vi "Process.vi"(8 "error in":errorcluster, 11 "SignalReceiver":refnum<class "SignalReceiver.lvclass">) -> (0 "error out":errorcluster, 3 "SignalReceiver out":refnum<class "SignalReceiver.lvclass">)   [LabVIEW 2020, in "ECU_Diagnose.lvlib" / "SignalReceiver.lvclass"]
doc: "---------------------------------------------------------------\nJKI State Machine Objects™\nhttp://jki.net/state-machine-objects/\nCopyright (C) 2005-2015, JKI <info@jki.net>\nALL RIGHTS RESERVEDJKI State Machine Objects (SMO) 1.0.0.5\nJKI - JKI\nCopyright (c) 2016, JKI"
uses:
  SignalReceiver.lvclass
  C:/Program Files (x86)/National Instruments/LabVIEW 2020/vi.lib/JKI/JKI SMO/SMO/SMO.lvclass
  <vilib>/JKI/JKI SMO/SMO/Typedefs/Parent Call--Enum.ctl
  <vilib>/JKI/JKI SMO/SMO/SMO.lvclass/SMO.ctl
  <vilib>/Platform/TimedLoop/XDataNode/timing_clust.ctl
  <vilib>/Platform/TimedLoop/XDataNode/nitl_modes.ctl
  <vilib>/Platform/TimedLoop/XDataNode/wakeup.ctl
  GlobalData_operation.ctl
  <vilib>/JKI/JKI SMO/SMO/Private/ReftoDVR--SMO.vi
  <vilib>/xnet/xnet.llb/XNET Create Session (Signal Input Waveform).vi
  <vilib>/xnet/xnet.llb/XNET Read (Signal Waveform) .vi
  <vilib>/Platform/TimedLoop/XDataNode/XDataNode.xnode
  <vilib>/JKI/JKI SMO/SMO/SMO.lvclass
  <vilib>/Platform/TimedLoop/XDataNode/XDNodeRunTimeDep.lvlib
  <resource>/objmgr/xnet.rc
panel:
  out "Waveform Chart":waveform(dbl)[](graph)=[{"t0"=timestamp(3761175860.010846 s since 1904-01-01), "dt"=0.001, "Y"=[0.0, 0.0, 0.0, 0.0, 0.0, 0.0, 0.0, 0.0, 0.0, 0.0, 0.0, 0.0, 0.0, 0.0, 0.0, 0.0, 0.0, 0.0, 0.0, 0.0, 0.0, 0.0, 0.0, 0.0, 0.0, 0.0, 0.0, 0.0, 0.0, 0.0, 0.0]}, {"t0"=timestamp(3761175860.010846 s since 1904-01-01), "dt"=0.001, "Y"=[8.0, 8.0, 8.0, 8.0, 8.0, 8.0, 8.0, 8.0, 8.0, 8.0, 9.0, 9.0, 9.0, 9.0, 9.0, 9.0, 9.0, 9.0, 9.0, 9.0, 10.0, 10.0, 10.0, 10.0, 10.0, 10.0, 10.0, 10.0, 10.0, 10.0, 11.0]}]
  out "StartStopCapture":bool
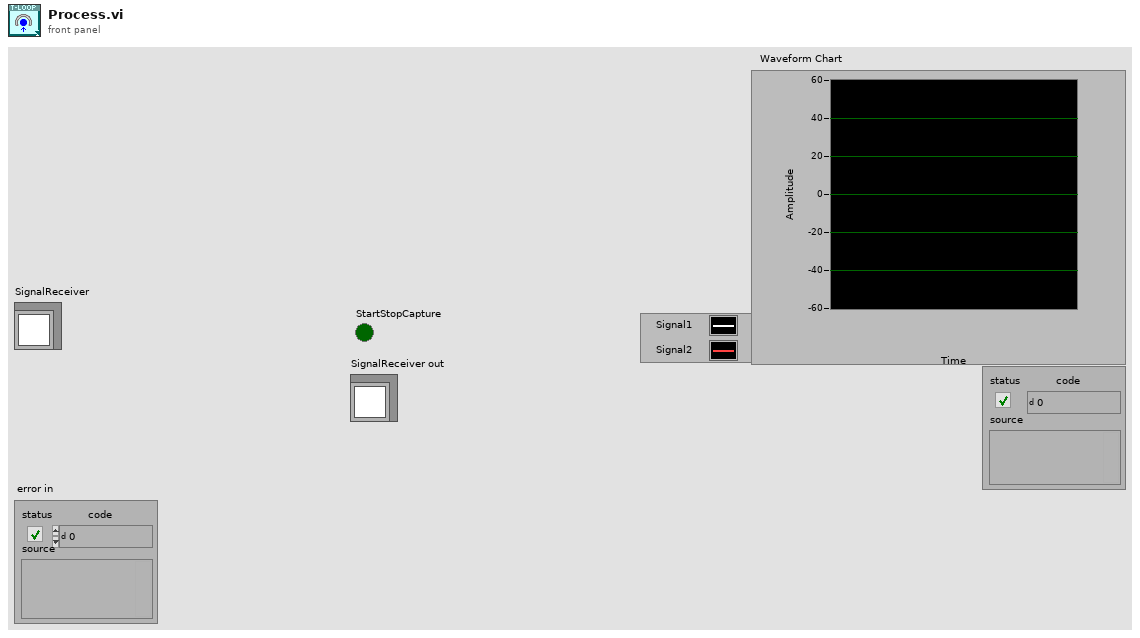
[diagram p1: front panel]
types:
  T1 = typedef "SMO.lvclass/Parent Call--Enum.ctl" = enum16{"Allows parent to run", "Does not request parent to run"}
  T2 = typedef "GlobalData_operation.ctl" = enum16{"idle", "read", "write", "clear", "init", "destroy"}
  T3 = typedef "XDNodeRunTimeDep.lvlib/timing_clust.ctl" = cluster{"Expected End [f-1]":u64, "Actual End [f-1]":u64, "Finished Late? [f-1]":bool, "Expected End [i-1]":u64, "Actual End [i-1]":u64, "Finished Late? [i-1]":bool, "Expected Start [i]":u64, "Actual Start [i]":u64, "Expected Start [f]":u64, "Actual Start [f]":u64, "Source Name":string, "Structure Name":string, "Period":i64, "Deadline":i64, "Offset":i64, "Start":i64, "Priority":i32, "Timeout":i32, "Mode":T4, "Wakeup Reason":T5, "Error":errorcluster, "Source Type":string, "Secondary Source Type":string, "Global End Time":u64, "Global Start Time":u64, "Frame Duration":u64, "Iteration Duration":u64, "Assigned CPU":i32, "I/O Scan Engine Mode":u32}
  T4 = typedef "XDNodeRunTimeDep.lvlib/nitl_modes.ctl" = enum32{"No Change", "Process missed periods, maintain original phase", "Discard missed periods, maintain original phase", "Process missed periods, ignore original phase", "Discard missed periods, ignore original phase"}
  T5 = typedef "XDNodeRunTimeDep.lvlib/wakeup.ctl" = enum32{"Normal", "Aborted", "Asynchronous wakeup", "Timing source error", "Timed loop error", "Timeout"}
  T6 = typedef "ECU_Diagnose.lvlib/SignalReceiver.lvclass/SignalArrySelecte.ctl" = cluster{"Port_No.":refnum<k21>, "XNET Signal":refnum<k21>[]}
  T7 = typedef "ECU_Diagnose.lvlib/SignalReceiver.lvclass/PrivateEvents--Cluster.ctl" = cluster{"AsyncMethod":refnum<user-event>, "Start_Stop":refnum<user-event>}
  T8 = typedef "SMO.lvclass/Protected Events.ctl" = cluster{"StopProcesses":refnum<user-event>, "AbortProcesses":refnum<user-event>, "Config Changed":refnum<user-event>, "Dependency":refnum<user-event>}
  T9 = typedef "ECU_Diagnose.lvlib/SignalReceiver.lvclass/PrivateEvents--SignalReceiver.Start_Stop.ctl" = bool
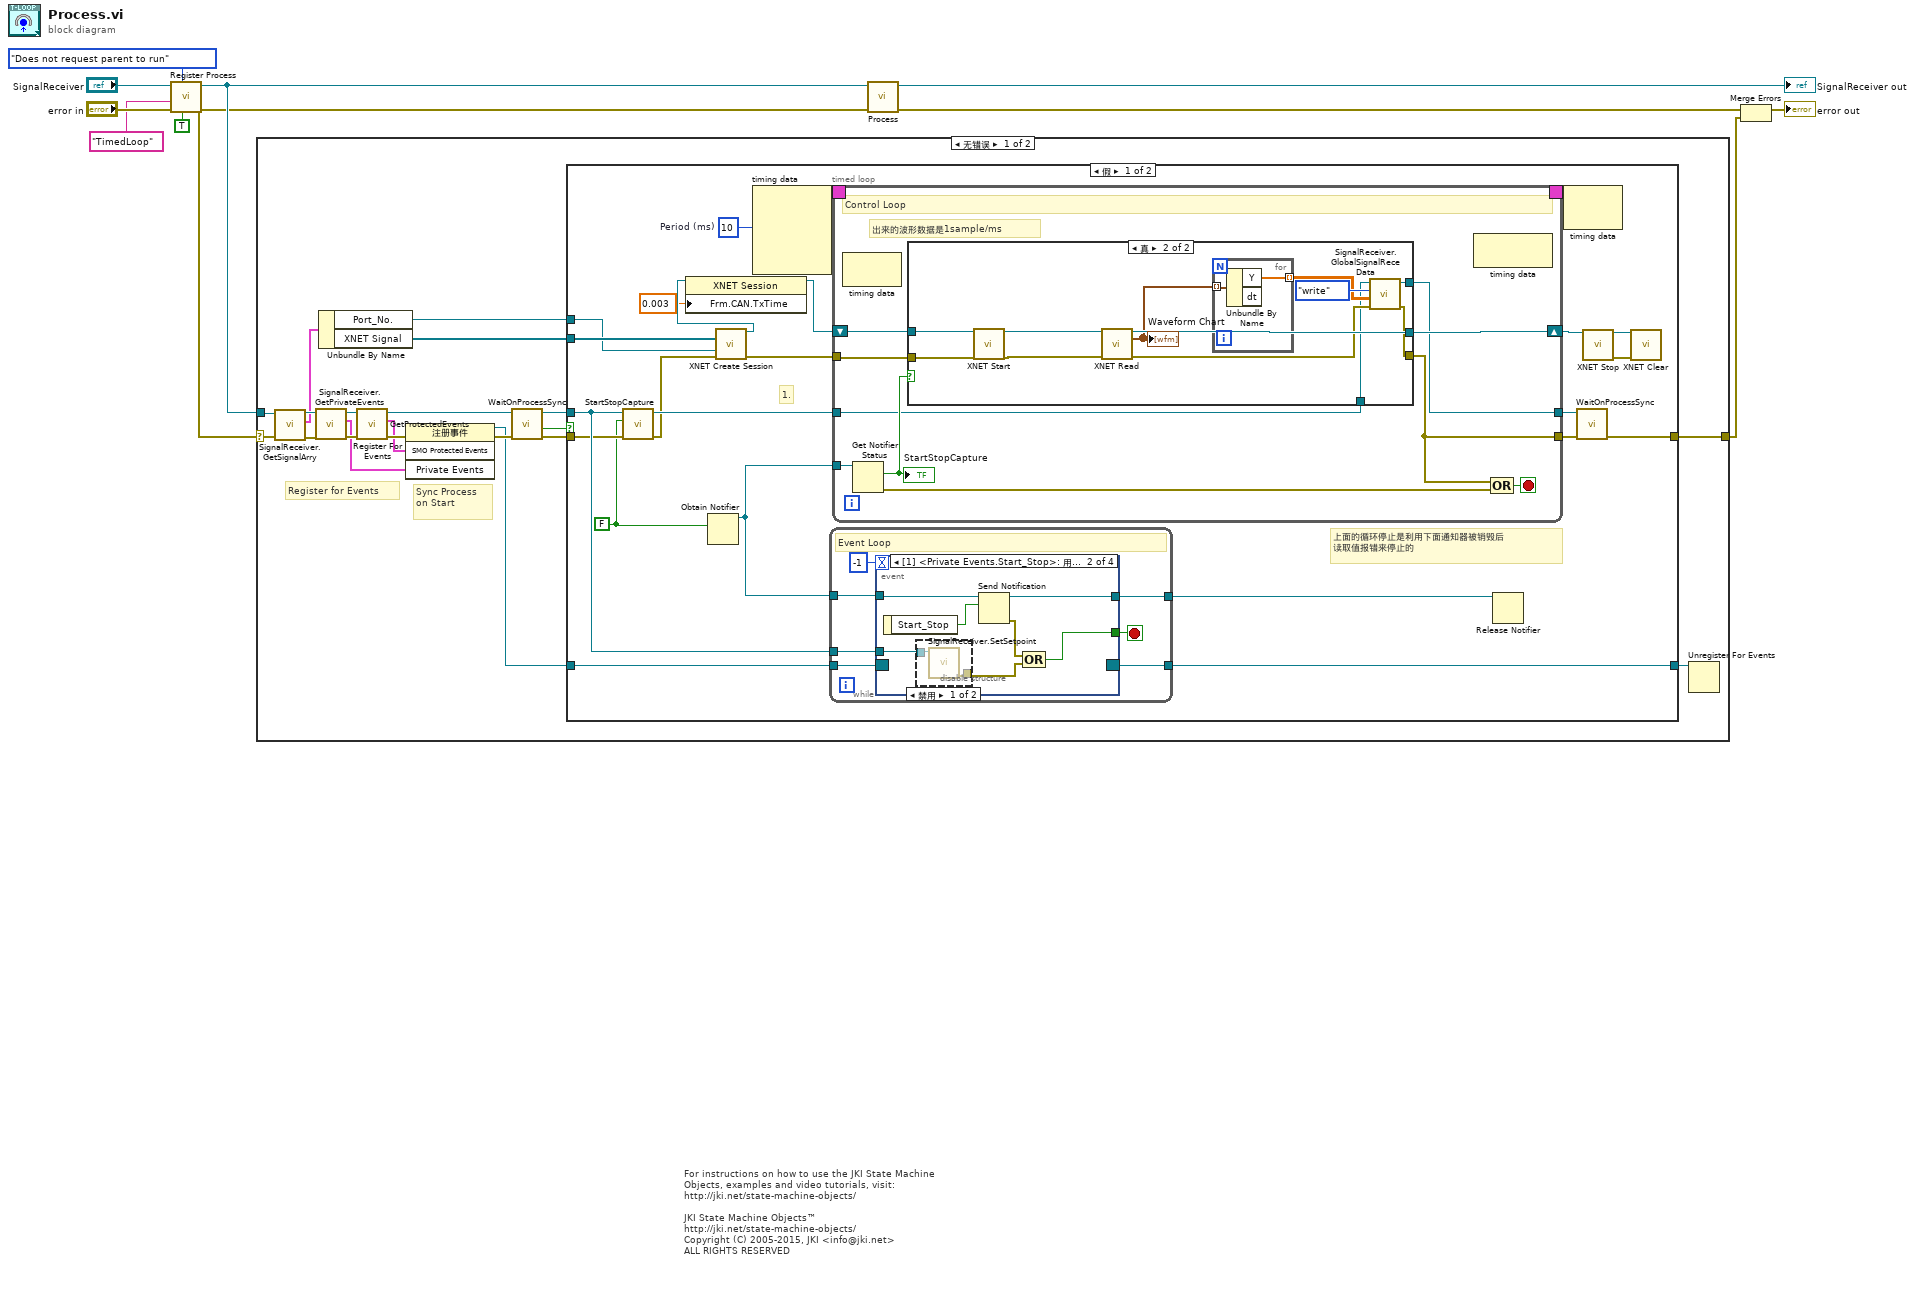
[diagram p0: block diagram]
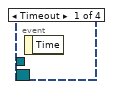
[diagram p2: hidden frame]
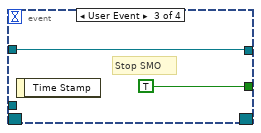
[diagram p4: hidden frame]
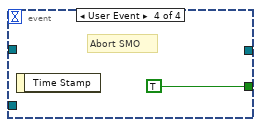
[diagram p5: hidden frame]
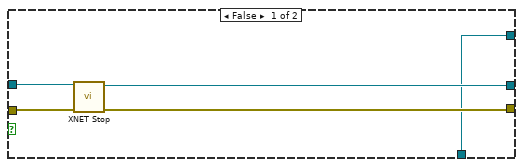
[diagram p6: hidden frame]
diagram:
  # "For instructions on how to use the JKI State Machine Objects, examples and video tutorials, visit:\nhttp://jki.net/state-machine-objects/\n\nJKI State Machine Objects™\nhttp://jki.net/state-machine-objects/\nCopyright (C) 2005-2015, JKI <info@jki.net>\nALL RIGHTS RESERVED"
  n1 = call <vilib>:"Register Process.vi"("Forces Self to Run (F)"=TRUE, "Parent Call"=Parent_Call--Enum."Does not request parent to run", "error in (no error)"="error in", "Process Name (optional)"="TimedLoop", "SMO"="SignalReceiver") -> ("error out"=w1:errorcluster, "SMO out"=w2:refnum<class "SignalReceiver.lvclass">)  [unwired: 5 in]
  n2 = case shown="无错误" w1 {
    selector: w1 -> [w16 w111]
    tunnel: w2 -> [w17 _]
    tunnel: [w23 w111] -> w6
    frame No Error {
      # "Sync Process\non Start"
      # "Register for Events"
      n3 = call "SignalReceiver.GetSignalArry.vi"("error in (no error)"=w16, "SignalReceiver"=w17) -> ("error out"=w15:errorcluster, "SignalArrySelect"=w14:T6, "SignalReceiver out"=w18:refnum<class "SignalReceiver.lvclass">)  [unwired: 7 in]
      n4 = call "SignalReceiver.GetPrivateEvents.vi"("error in (no error)"=w15, "SignalReceiver"=w18) -> ("error out"=w20:errorcluster, "Private Events"=w19:T7, "SignalReceiver out"=w21:refnum<class "SignalReceiver.lvclass">)  [unwired: 7 in]
      n5 = Unbundle By Name(w14) -> ("Port_No."=w12:refnum<k21>, "XNET Signal"=w13:refnum<k21>[])
      n6 = call <vilib>:"GetProtectedEvents.vi"("error in (no error)"=w20, "SMO"=w21) -> ("error out"=w26:errorcluster, "SMO Protected Events"=w25:T8, "SMO out"=w27:refnum<class "SignalReceiver.lvclass">)  [unwired: 7 in]
      n7 = register-events(error in=w26, w25, w19) -> (reference out=w24:refnum<event-registration>, error out=w28:errorcluster)  [unwired: 1 in]
      n8 = call <vilib>:"WaitOnProcessSync.vi"("error in (no error)"=w28, "SMO"=w27) -> ("error out"=w30:errorcluster, "Don't run?"=w31:bool, "SMO out"=w29:refnum<class "SignalReceiver.lvclass">)  [unwired: 7 in]
      n9 = case shown="假" w31 {
        tunnel: w30 -> [w43 w109]
        tunnel: w29 -> [w44 _]
        tunnel: w24 -> [w49 w110]
        tunnel: [w50 w109] -> w23
        tunnel: [w48 w110] -> w22
        tunnel: w13 -> [w39 _]
        tunnel: w12 -> [w38 _]
        frame False {
          w41 = FALSE
          w53 = i64 10  # Period (ms)
          # "上面的循环停止是利用下面通知器被销毁后\n读取值报错来停止的"
          # "1."
          n10 = call "StartStopCapture.vi"("error in (no error)"=w43, "StartStopCapture"=w41, "SignalReceiver"=w44) -> ("error out"=w40:errorcluster, "SignalReceiver out"=w42:refnum<class "SignalReceiver.lvclass">)  [unwired: 7 in]
          n11 = Obtain Notifier(notification data type=w41) -> (notifier out=w47:refnum<notifier>)  [unwired: 3 in, 2 out]
          n12 = call-poly <vilib>:"XNET Create Session.vi"("signal list"=w39, "interface"=w38, "error in (no error)"=w40) -> ("session out"=w34:refnum<k21>, "error out"=w45:errorcluster)  [unwired: 11 out]
          n13 = property class="XNET Session"(reference=w34, "Frm.CAN.TxTime"=0.003 ("Frame:CAN:Transmit Time")) -> (reference out=w32:refnum<k21>)  [unwired: 1 in, 1 out]
          n14 = node-c288(w53) -> (w55:T3)  [unwired: 3 in]
          n15 = while {
            tunnel: w49 -> [w61]
            tunnel: [w60] -> w48
            tunnel: w44 -> [w58]
            tunnel: w47 -> [w57]
            tunnel: [w56] -> w46
            stop <- w59 stop-if-true
            # "Event Loop"
            n16 = event shown="[1] <Private Events.Start_Stop>: 用户事件" {
              selector: w61 -> [_ _ _ _]
              dyn-events: [_ _ _ _] -> w60
              timeout: -1 -> [_ _ _ _]
              tunnel: [_ w66 TRUE TRUE] -> w59
              tunnel: w58 -> [_ w69 _ _]
              tunnel: w57 -> [_ w65 w72 _]
              tunnel: [_ w64 w72 _] -> w56
              event Timeout {
                n17 = event-data() -> ()  [unwired: 1 in, 1 out]
              }
              event User Event {
                n18 = event-data() -> ("Start_Stop"=w63:T9)  [unwired: 1 in]
                n19 = disable-structure shown="禁用" {
                  disable-tunnel: w69 -> [w71 _]
                  disable-tunnel: [w70 _] -> w68
                  frame Disabled {
                    n20 = call "SignalReceiver.SetSetpoint.vi"("SignalReceiver"=w71) -> ("error out"=w70:errorcluster)  [unwired: 9 in, 1 out]
                  }
                  frame Enabled {
                  }
                }
                n21 = Send Notification(notification=w63, notifier=w65) -> (notifier out=w64:refnum<notifier>, error out=w67:errorcluster)  [unwired: 1 in]
                n22 = Compound Arithmetic op=OR(w67, w68) -> (w66:bool)
              }
              event User Event {
                # "Stop SMO"
                n23 = event-data() -> ()  [unwired: 1 in, 1 out]
              }
              event User Event {
                # "Abort SMO"
                n24 = event-data() -> ()  [unwired: 1 in, 1 out]
              }
            }
          }
          n25 = timed-loop {
            timing: w55 -> [_]
            timing-out: [_] -> w54
            tunnel: w42 -> [w76]
            tunnel: [w75] -> w52
            tunnel: [w77] -> w51
            tunnel: w47 -> [w83]
            tunnel: w45 -> [w81]
            shift-right: [w78] -> w37
            shift-left: w32 -> [w82]
            stop <- w84 stop-if-true
            # "出来的波形数据是1sample/ms"
            # "Control Loop"
            n26 = node-c288() -> ()  [unwired: 1 in, 1 out]
            n27 = Get Notifier Status(notifier=w83) -> (current notification=w79:bool, error out=w80:errorcluster)  [unwired: 1 in, 3 out]
            "StartStopCapture" <- w79
            n28 = case shown="真" w79 {
              tunnel: w82 -> [w89 w90]
              tunnel: w81 -> [w88 w100]
              tunnel: [w87 w99] -> w78
              tunnel: [w86 w95] -> w77
              tunnel: w76 -> [w85 w93]
              tunnel: [w85 w92] -> w75
              frame False {
                n29 = call <vilib>:"XNET Stop.vi"("session in"=w89, "error in (no error)"=w88) -> ("session out"=w87:refnum<k21>, "error out"=w86:errorcluster)  [unwired: 12 in]
              }
              frame True {
                n30 = call <vilib>:"XNET Start.vi"("session in"=w90) -> ("session out"=w91:refnum<k21>)  [unwired: 13 in, 1 out]
                n31 = call-poly <vilib>:"XNET Read.vi"("session in"=w91, "error in (no error)"=w100) -> ("session out"=w99:refnum<k21>, "data"=w98:waveform(dbl)[], "error out"=w96:errorcluster)  [unwired: 11 out]
                "Waveform Chart" <- w98
                n32 = for {
                  tunnel: w98 -> [w102] mode=indexing
                  tunnel: [w101] -> w94 mode=indexing
                  n33 = Unbundle By Name(w102) -> ("Y"=w101:dbl[])  [unwired: 1 out]
                }
                n34 = call "SignalReceiver.GlobalSignalReceData.vi"("error in (no error)"=w96, "SignalDatIn"=w94, "operation"=GlobalData_operation."write", "SignalReceiver"=w93) -> ("error out"=w95:errorcluster, "SignalReceiver out"=w92:refnum<class "SignalReceiver.lvclass">)  [unwired: 4 in, 2 out]
              }
            }
            n35 = node-c288() -> ()  [unwired: 1 in, 1 out]
            n36 = Compound Arithmetic op=OR(w77, w80) -> (w84:bool)
          }
          n37 = Release Notifier(notifier=w46) -> ()  [unwired: 2 in, 3 out]
          n38 = node-c288(w54) -> ()  [unwired: 1 out]
          n39 = call <vilib>:"WaitOnProcessSync.vi"("error in (no error)"=w51, "SMO"=w52) -> ("error out"=w50:errorcluster)  [unwired: 7 in, 2 out]
          n40 = call <vilib>:"XNET Stop.vi"("session in"=w37) -> ("session out"=w35:refnum<k21>, "error out"=w36:errorcluster)  [unwired: 13 in]
          n41 = call <vilib>:"XNET Clear.vi"("session in"=w35, "error in (no error)"=w36) -> ()  [unwired: 13 in, 1 out]
        }
        frame True {
        }
      }
      n42 = Unregister For Events(event registration refnum=w22) -> ()  [unwired: 1 in, 1 out]
    }
    frame Error {
    }
  }
  n43 = call-parent "Process.vi"("error in"=w1, "SMO"=w2) -> ("error out"=w7:errorcluster, "SMO out"=→"SignalReceiver out":refnum<class "SignalReceiver.lvclass">)  [unwired: 8 in]
  n44 = Merge Errors(w7, w6) -> (→"error out":errorcluster)
